vi "Set64PinPGAXRay.vi"(11 "Pattern":T1) -> (3 "X-Ray PGA":T3)   [LabVIEW 2012, in "Virtual-PGA.lvlib"]
doc: "This VI sets the indicators for the X-ray indicator of the PGA."
uses:
  Virtual-PGA.lvlib
  Controls/64PinPGAXRay.ctl
  Controls/Pattern.ctl
  Controls/Input.ctl
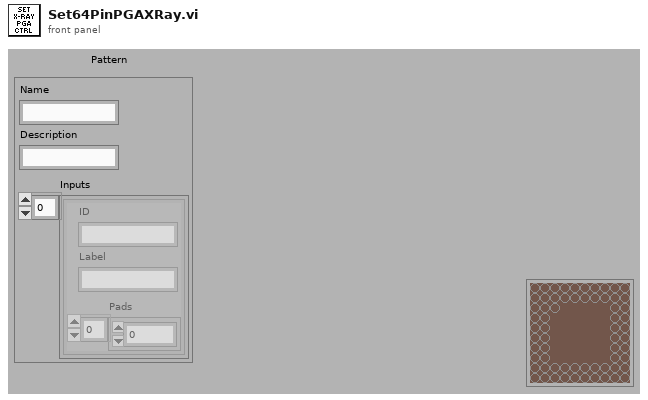
[diagram p1: front panel]
types:
  T1 = typedef "Virtual-PGA.lvlib/Pattern.ctl" = cluster{"Name":string, "Description":string, "Inputs":T2[]}
  T2 = typedef "Virtual-PGA.lvlib/Input.ctl" = cluster{"ID":string, "Label":string, "Pads":u32[]}
  T3 = typedef "Virtual-PGA.lvlib/64PinPGAXRay.ctl" = cluster{"Pin 1":bool, "Pin 2":bool, "Pin 3":bool, "Pin 53":bool, "Pin 64":bool, "Pin 50":bool, "Pin 62":bool, "Pin 60":bool, "Pin 58":bool, "Pin 56":bool, "Pin 42":bool, "Pin 44":bool, "Pin 48":bool, "Pin 46":bool, "Pin 51":bool, "Pin 40":bool, "Pin 37":bool, "Pin 30":bool, "Pin 26":bool, "Pin 32":bool, "Pin 28":bool, "Pin 34":bool, "Pin 24":bool, "Pin 31":bool, "Pin 21":bool, "Pin 18":bool, "Pin 19":bool, "Pin 16":bool, "Pin 14":bool, "Pin 12":bool, "Pin 10":bool, "Pin 8":bool, "Pin 5":bool, "Pin 63":bool, "Pin 61":bool, "Pin 59":bool, "Pin 57":bool, "Pin 55":bool, "Pin 54":bool, "Pin 52":bool, "Pin 65":bool, "Pin 29":bool, "Pin 27":bool, "Pin 25":bool, "Pin 23":bool, "Pin 22":bool, "Pin 20":bool, "Pin 33":bool, "Pin 35":bool, "Pin 36":bool, "Pin 38":bool, "Pin 39":bool, "Pin 41":bool, "Pin 43":bool, "Pin 45":bool, "Pin 47":bool, "Pin 49":bool, "Pin 17":bool, "Pin 15":bool, "Pin 13":bool, "Pin 11":bool, "Pin 9":bool, "Pin 7":bool, "Pin 6":bool, "Pin 4":bool}
  T4 = cluster{"Y1":bool, "Y2":bool, "Y3":bool, "Y4":bool}[]
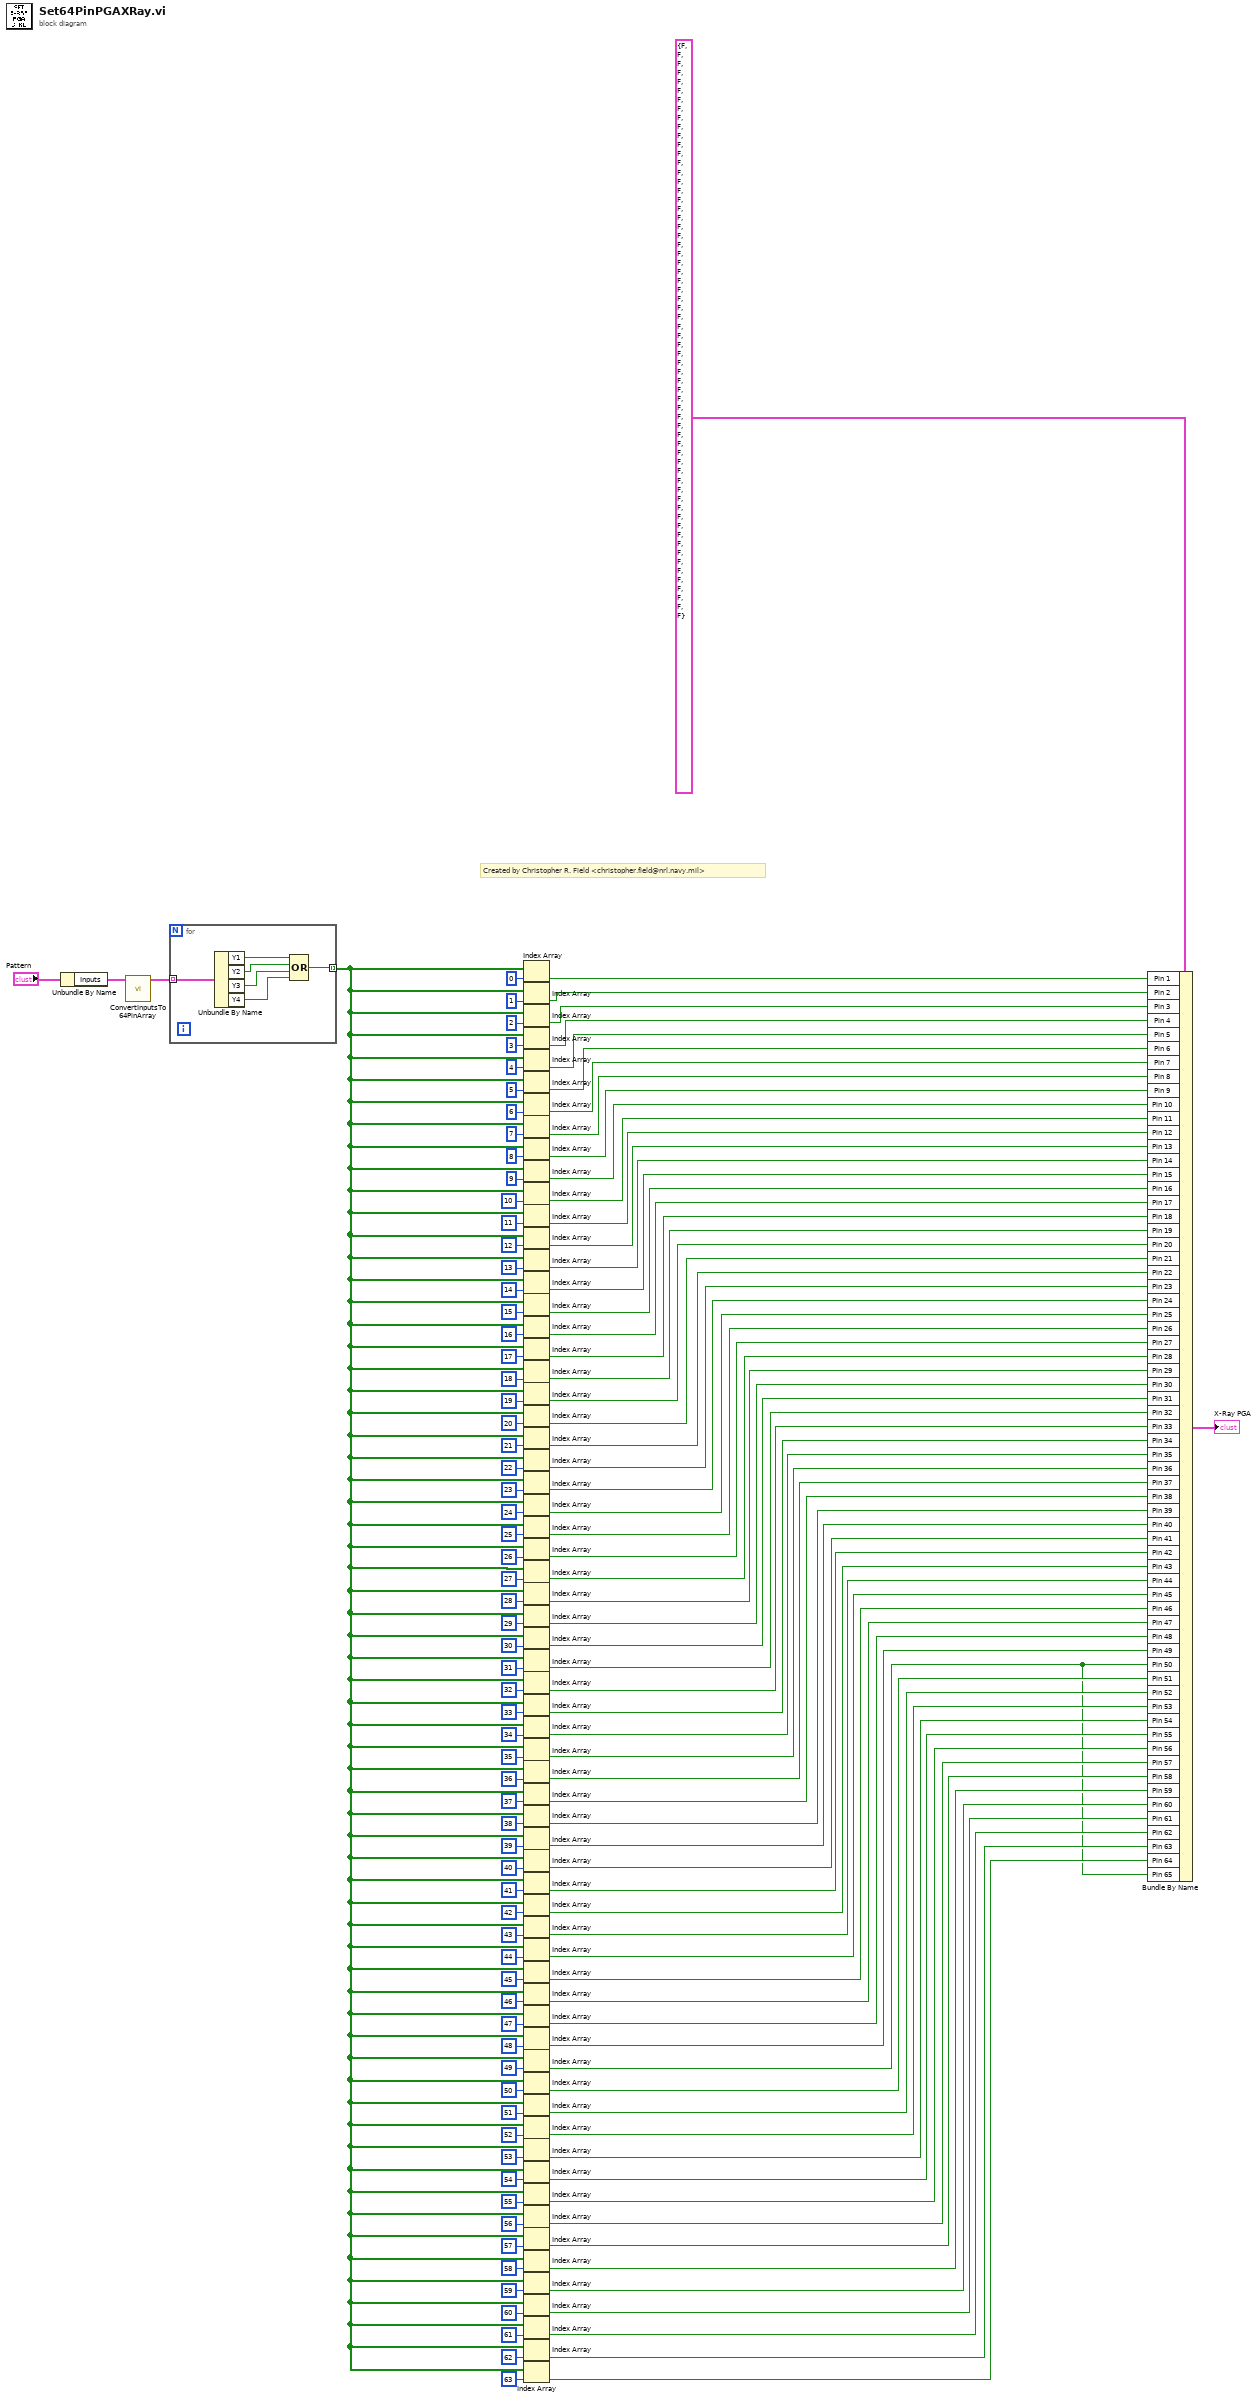
[diagram p0: block diagram]
diagram:
  # "Created by Christopher R. Field <christopher.field@nrl.navy.mil>"
  n1 = Unbundle By Name("Pattern") -> ("Inputs"=w6:T2[])
  n2 = call "ConvertInputsTo64PinArray.vi"("Inputs"=w6) -> ("64-Pin Array"=w5:T4)  [unwired: 10 in]
  n3 = for {
    tunnel: [w136] -> w2 mode=indexing
    tunnel: w5 -> [w135] mode=indexing
    n4 = Unbundle By Name(w135) -> ("Y1"=w140:bool, "Y2"=w139:bool, "Y3"=w138:bool, "Y4"=w137:bool)
    n5 = Compound Arithmetic op=OR(w140, w139, w138, w137) -> (w136:bool)
  }
  n6 = Index Array(array=w2, index=0) -> (element=w132:bool)
  n7 = Index Array(array=w2, index=1) -> (element=w130:bool)
  n8 = Index Array(array=w2, index=2) -> (element=w128:bool)
  n9 = Index Array(array=w2, index=3) -> (element=w126:bool)
  n10 = Index Array(array=w2, index=4) -> (element=w124:bool)
  n11 = Index Array(array=w2, index=5) -> (element=w122:bool)
  n12 = Index Array(array=w2, index=6) -> (element=w120:bool)
  n13 = Index Array(array=w2, index=7) -> (element=w62:bool)
  n14 = Index Array(array=w2, index=8) -> (element=w61:bool)
  n15 = Index Array(array=w2, index=9) -> (element=w60:bool)
  n16 = Index Array(array=w2, index=10) -> (element=w59:bool)
  n17 = Index Array(array=w2, index=11) -> (element=w58:bool)
  n18 = Index Array(array=w2, index=12) -> (element=w57:bool)
  n19 = Index Array(array=w2, index=13) -> (element=w56:bool)
  n20 = Index Array(array=w2, index=14) -> (element=w55:bool)
  n21 = Index Array(array=w2, index=15) -> (element=w54:bool)
  n22 = Index Array(array=w2, index=16) -> (element=w53:bool)
  n23 = Index Array(array=w2, index=17) -> (element=w52:bool)
  n24 = Index Array(array=w2, index=18) -> (element=w51:bool)
  n25 = Index Array(array=w2, index=19) -> (element=w50:bool)
  n26 = Index Array(array=w2, index=20) -> (element=w49:bool)
  n27 = Index Array(array=w2, index=21) -> (element=w48:bool)
  n28 = Index Array(array=w2, index=22) -> (element=w47:bool)
  n29 = Index Array(array=w2, index=23) -> (element=w46:bool)
  n30 = Index Array(array=w2, index=24) -> (element=w45:bool)
  n31 = Index Array(array=w2, index=25) -> (element=w44:bool)
  n32 = Index Array(array=w2, index=26) -> (element=w43:bool)
  n33 = Index Array(array=w2, index=27) -> (element=w42:bool)
  n34 = Index Array(array=w2, index=28) -> (element=w41:bool)
  n35 = Index Array(array=w2, index=29) -> (element=w40:bool)
  n36 = Index Array(array=w2, index=30) -> (element=w39:bool)
  n37 = Index Array(array=w2, index=31) -> (element=w38:bool)
  n38 = Index Array(array=w2, index=32) -> (element=w37:bool)
  n39 = Index Array(array=w2, index=33) -> (element=w36:bool)
  n40 = Index Array(array=w2, index=34) -> (element=w35:bool)
  n41 = Index Array(array=w2, index=35) -> (element=w34:bool)
  n42 = Index Array(array=w2, index=36) -> (element=w33:bool)
  n43 = Index Array(array=w2, index=37) -> (element=w32:bool)
  n44 = Index Array(array=w2, index=38) -> (element=w31:bool)
  n45 = Index Array(array=w2, index=39) -> (element=w30:bool)
  n46 = Index Array(array=w2, index=40) -> (element=w29:bool)
  n47 = Index Array(array=w2, index=41) -> (element=w28:bool)
  n48 = Index Array(array=w2, index=42) -> (element=w27:bool)
  n49 = Index Array(array=w2, index=43) -> (element=w26:bool)
  n50 = Index Array(array=w2, index=44) -> (element=w25:bool)
  n51 = Index Array(array=w2, index=45) -> (element=w24:bool)
  n52 = Index Array(array=w2, index=46) -> (element=w23:bool)
  n53 = Index Array(array=w2, index=47) -> (element=w22:bool)
  n54 = Index Array(array=w2, index=48) -> (element=w21:bool)
  n55 = Index Array(array=w2, index=49) -> (element=w3:bool)
  n56 = Index Array(array=w2, index=50) -> (element=w20:bool)
  n57 = Index Array(array=w2, index=51) -> (element=w19:bool)
  n58 = Index Array(array=w2, index=52) -> (element=w18:bool)
  n59 = Index Array(array=w2, index=53) -> (element=w17:bool)
  n60 = Index Array(array=w2, index=54) -> (element=w16:bool)
  n61 = Index Array(array=w2, index=55) -> (element=w15:bool)
  n62 = Index Array(array=w2, index=56) -> (element=w14:bool)
  n63 = Index Array(array=w2, index=57) -> (element=w13:bool)
  n64 = Index Array(array=w2, index=58) -> (element=w12:bool)
  n65 = Index Array(array=w2, index=59) -> (element=w11:bool)
  n66 = Index Array(array=w2, index=60) -> (element=w10:bool)
  n67 = Index Array(array=w2, index=61) -> (element=w9:bool)
  n68 = Index Array(array=w2, index=62) -> (element=w8:bool)
  n69 = Index Array(array=w2, index=63) -> (element=w4:bool)
  n70 = Bundle By Name(cluster=T3 {"Pin 1"=FALSE, "Pin 2"=FALSE, "Pin 3"=FALSE, "Pin 53"=FALSE, "Pin 64"=FALSE, "Pin 50"=FALSE, "Pin 62"=FALSE, "Pin 60"=FALSE, "Pin 58"=FALSE, "Pin 56"=FALSE, "Pin 42"=FALSE, "Pin 44"=FALSE, "Pin 48"=FALSE, "Pin 46"=FALSE, "Pin 51"=FALSE, "Pin 40"=FALSE, "Pin 37"=FALSE, "Pin 30"=FALSE, "Pin 26"=FALSE, "Pin 32"=FALSE, "Pin 28"=FALSE, "Pin 34"=FALSE, "Pin 24"=FALSE, "Pin 31"=FALSE, "Pin 21"=FALSE, "Pin 18"=FALSE, "Pin 19"=FALSE, "Pin 16"=FALSE, "Pin 14"=FALSE, "Pin 12"=FALSE, "Pin 10"=FALSE, "Pin 8"=FALSE, "Pin 5"=FALSE, "Pin 63"=FALSE, "Pin 61"=FALSE, "Pin 59"=FALSE, "Pin 57"=FALSE, "Pin 55"=FALSE, "Pin 54"=FALSE, "Pin 52"=FALSE, "Pin 65"=FALSE, "Pin 29"=FALSE, "Pin 27"=FALSE, "Pin 25"=FALSE, "Pin 23"=FALSE, "Pin 22"=FALSE, "Pin 20"=FALSE, "Pin 33"=FALSE, "Pin 35"=FALSE, "Pin 36"=FALSE, "Pin 38"=FALSE, "Pin 39"=FALSE, "Pin 41"=FALSE, "Pin 43"=FALSE, "Pin 45"=FALSE, "Pin 47"=FALSE, "Pin 49"=FALSE, "Pin 17"=FALSE, "Pin 15"=FALSE, "Pin 13"=FALSE, "Pin 11"=FALSE, "Pin 9"=FALSE, "Pin 7"=FALSE, "Pin 6"=FALSE, "Pin 4"=FALSE} ("X-Ray PGA"), "Pin 1"=w132, "Pin 2"=w130, "Pin 3"=w128, "Pin 4"=w126, "Pin 5"=w124, "Pin 6"=w122, "Pin 7"=w120, "Pin 8"=w62, "Pin 9"=w61, "Pin 10"=w60, "Pin 11"=w59, "Pin 12"=w58, "Pin 13"=w57, "Pin 14"=w56, "Pin 15"=w55, "Pin 16"=w54, "Pin 17"=w53, "Pin 18"=w52, "Pin 19"=w51, "Pin 20"=w50, "Pin 21"=w49, "Pin 22"=w48, "Pin 23"=w47, "Pin 24"=w46, "Pin 25"=w45, "Pin 26"=w44, "Pin 27"=w43, "Pin 28"=w42, "Pin 29"=w41, "Pin 30"=w40, "Pin 31"=w39, "Pin 32"=w38, "Pin 33"=w37, "Pin 34"=w36, "Pin 35"=w35, "Pin 36"=w34, "Pin 37"=w33, "Pin 38"=w32, "Pin 39"=w31, "Pin 40"=w30, "Pin 41"=w29, "Pin 42"=w28, "Pin 43"=w27, "Pin 44"=w26, "Pin 45"=w25, "Pin 46"=w24, "Pin 47"=w23, "Pin 48"=w22, "Pin 49"=w21, "Pin 50"=w3, "Pin 51"=w20, "Pin 52"=w19, "Pin 53"=w18, "Pin 54"=w17, "Pin 55"=w16, "Pin 56"=w15, "Pin 57"=w14, "Pin 58"=w13, "Pin 59"=w12, "Pin 60"=w11, "Pin 61"=w10, "Pin 62"=w9, "Pin 63"=w8, "Pin 64"=w4, "Pin 65"=w3) -> (→"X-Ray PGA":T3)
